vi "Run.vi"(8 "error in (no error)":errorcluster caption="entrée d'erreur (pas d'erreur)", 9 "y_score":string[][](array[string]), 10 "y_true":string[][](array[string]), 11 "Average_Precision_Score.lvclass":refnum<class "Average_Precision_Score.lvclass">) -> (0 "error out":errorcluster caption="sortie d'erreur", 2 "String Data":string, 3 "Average_Precision_Score.lvclass":refnum<class "Average_Precision_Score.lvclass">)   [LabVIEW 2020, in "Average_Precision_Score.lvclass"]
doc: "Returns :\n\n- average_precision : float"
uses:
  Average_Precision_Score.lvclass
  Average_Precision_Score.lvclass/Average_Precision_Score.ctl
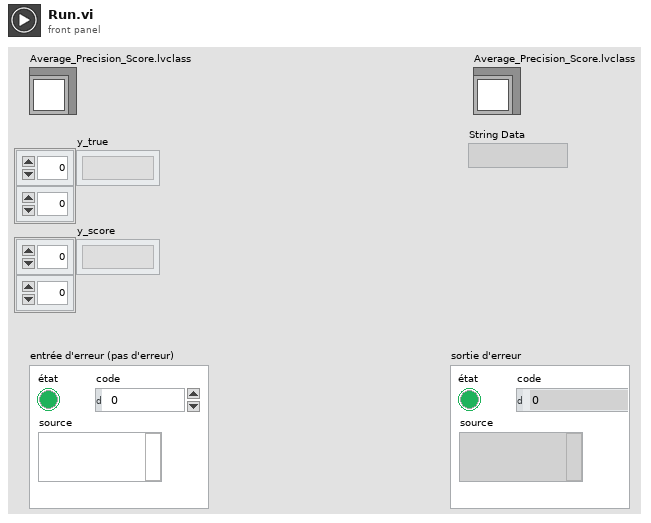
[diagram p1: front panel]
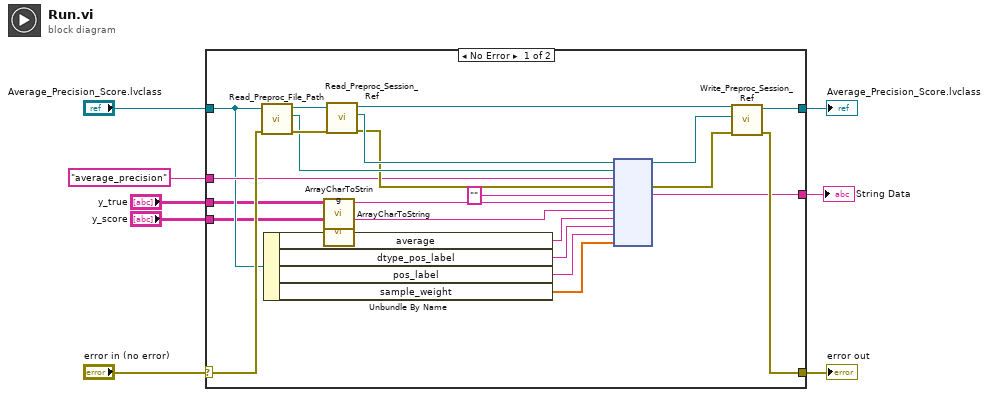
[diagram p0: block diagram]
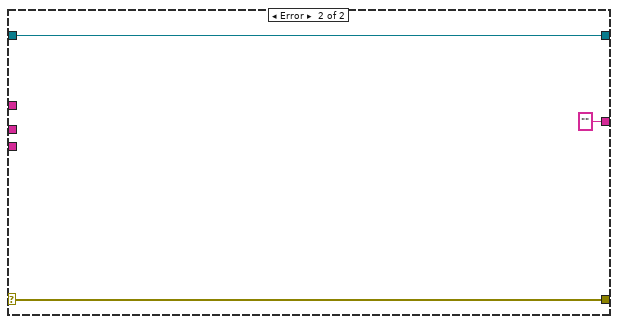
[diagram p2: hidden frame]
diagram:
  n1 = case shown="No Error" "error in (no error)" {
    selector: "error in (no error)" -> [w20 w34]
    tunnel: [w21 w34] -> w7
    tunnel: [w22 w33] -> w5
    tunnel: "Average_Precision_Score.lvclass" -> [w17 w33]
    tunnel: "average_precision" -> [w19 _]
    tunnel: [w18 ""] -> w4
    tunnel: "y_true" -> [w12 _]
    tunnel: "y_score" -> [w11 _]
    frame No Error {
      n2 = call-dynamic "Read_Preproc_File_Path.vi"("error in (no error)"=w20, "Python in"=w17) -> ("error out"=w30:errorcluster, "File_Path"=w29:path, "Python out"=w31:refnum<class "Average_Precision_Score.lvclass">)  [unwired: 7 in]
      n3 = Unbundle By Name(w17) -> ("average"=w16:string, "dtype_pos_label"=w15:string, "pos_label"=w14:string, "sample_weight"=w13:dbl[])
      n4 = call "ArrayCharToString.vi"("TAB"=w12) -> ("Instruction"=w10:string)  [unwired: 10 in]
      n5 = call "ArrayCharToString.vi"("TAB"=w11) -> ("Instruction"=w9:string)  [unwired: 10 in]
      n6 = call-dynamic "Read_Preproc_Session_Ref.vi"("error in (no error)"=w30, "Python in"=w31) -> ("error out"=w27:errorcluster, "Session_ref"=w28:refnum<k35>, "Python out"=w26:refnum<class "Average_Precision_Score.lvclass">)  [unwired: 7 in]
      n7 = node(w28, w29, w19, w27, "", w10, w9, w16, w15, w14, w13) -> (w24:refnum<k35>, w25:errorcluster, w18:string)  [unwired: 6 in, 2 out]
      n8 = call-dynamic "Write_Preproc_Session_Ref.vi"("error in (no error)"=w25, "Session_ref"=w24, "Python in"=w26) -> ("error out"=w21:errorcluster, "Python out"=w22:refnum<class "Average_Precision_Score.lvclass">)  [unwired: 7 in]
    }
    frame Error {
    }
  }
  "error out" <- w7
  "Average_Precision_Score.lvclass" <- w5
  "String Data" <- w4
